vi "ConfigurationSubVI.vi"(8 "error in (no error)":errorcluster, 10 "Sim? Cluster":T3, 11 "Channels Cluster":T2) -> (0 "error out":errorcluster, 3 "Data Cluster":T1)   [LabVIEW 2017]
doc: "Calls SubVIs configuring DAQ tasks."
uses:
  Controls/ShiftRegisterCluster.ctl
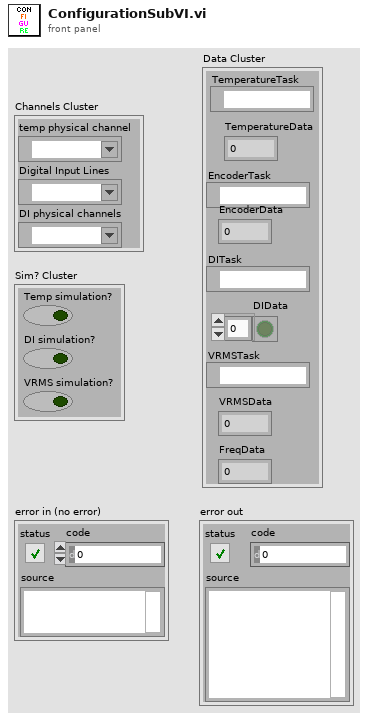
[diagram p1: front panel]
types:
  T1 = typedef "ShiftRegisterCluster.ctl" = cluster{"TemperatureTask":refnum<k21>, "TemperatureData":dbl, "EncoderTask":refnum<k21>, "EncoderData":dbl, "DITask":refnum<k21>, "DIData":bool[], "VRMSTask":refnum<k21>, "VRMSData":dbl, "FreqData":dbl}
  T2 = cluster{"temp physical channel":tag, "Digital Input Lines":tag, "DI physical channels":tag}
  T3 = cluster{"Temp simulation?":bool, "DI simulation?":bool, "VRMS simulation?":bool}
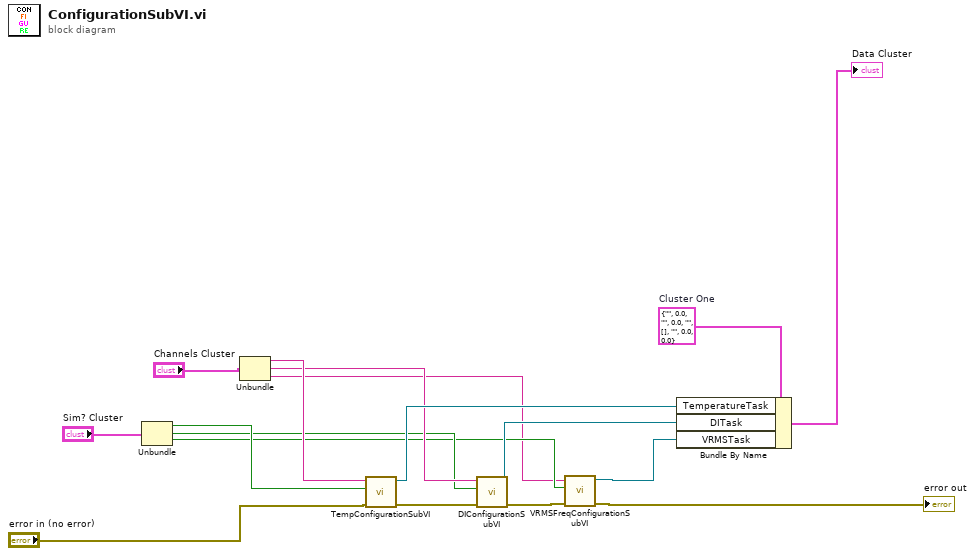
[diagram p0: block diagram]
diagram:
  w12 = T1 {"TemperatureTask"="", "TemperatureData"=0.0, "EncoderTask"="", "EncoderData"=0.0, "DITask"="", "DIData"=[], "VRMSTask"="", "VRMSData"=0.0, "FreqData"=0.0}  # Cluster One
  n1 = Unbundle("Sim? Cluster") -> ("Temp simulation?"=w17:bool, "DI simulation?"=w6:bool, "VRMS simulation?"=w5:bool)
  n2 = Unbundle("Channels Cluster") -> ("temp physical channel"=w11:tag, "Digital Input Lines"=w9:tag, "DI physical channels"=w4:tag)
  n3 = call "TempConfigurationSubVI.vi"("error in"="error in (no error)", "Sim?"=w17, "physical channels"=w11) -> ("error out"=w7:errorcluster, "task out"=w10:refnum<k21>)  [unwired: 7 in]
  n4 = call "DIConfigurationSubVI.vi"("error in"=w7, "Sim?"=w6, "Input Lines"=w9) -> ("error out"=w3:errorcluster, "task out"=w14:refnum<k21>)  [unwired: 7 in]
  n5 = call "VRMSFreqConfigurationSubVI.vi"("error in"=w3, "Sim?"=w5, "physical channel"=w4) -> ("error out"=→"error out":errorcluster, "task out"=w1:refnum<k21>)  [unwired: 7 in]
  n6 = Bundle By Name(cluster=w12, "TemperatureTask"=w10, "DITask"=w14, "VRMSTask"=w1) -> (→"Data Cluster":T1)
